vi "Output.vi"(10 "input valid":bool, 11 "input data":bool[](array[boolean])) -> (2 "output valid":bool, 3 "output data":fxp<+/-,20,5>)   [LabVIEW 2011]
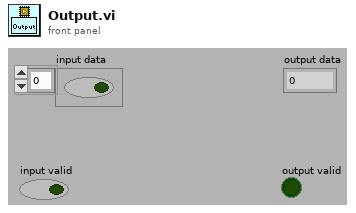
[diagram p1: front panel]
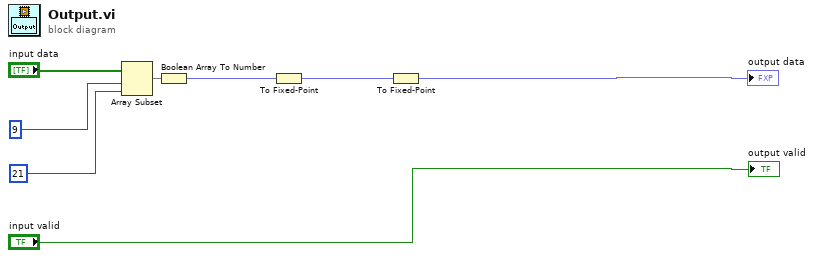
[diagram p0: block diagram]
diagram:
  n1 = Array Subset(array="input data", index=9 ("output index"), length=21 ("output length")) -> (w4:bool[])
  n2 = Boolean Array To Number ("KOutCvt")(Boolean array=w4) -> (number=w8:fxp<+/-,21,5>)
  n3 = To Fixed-Point ("KOutCast")(number=w8) -> (fixed-point=w3:fxp<+/-,20,5>)  [unwired: 1 in]
  n4 = To Fixed-Point ("KOut2FXP")(number=w3) -> (fixed-point=→"output data":fxp<+/-,20,5>)  [unwired: 1 out]
  "output valid" <- "input valid"
